vi "Untitled 1.vi"() -> ()   [LabVIEW 2025]
panel:
  out "Boolean 2":bool
  in  "Sair":bool
  out "Contador":dbl format="%#_2f"
  out "Boolean":bool
  in  "Pausar":bool
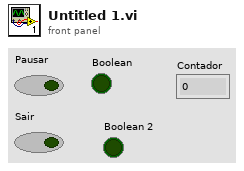
[diagram p1: front panel]
types:
  T1 = enum16{"Incializar", "Executar ", "Pausar", "Sair"}
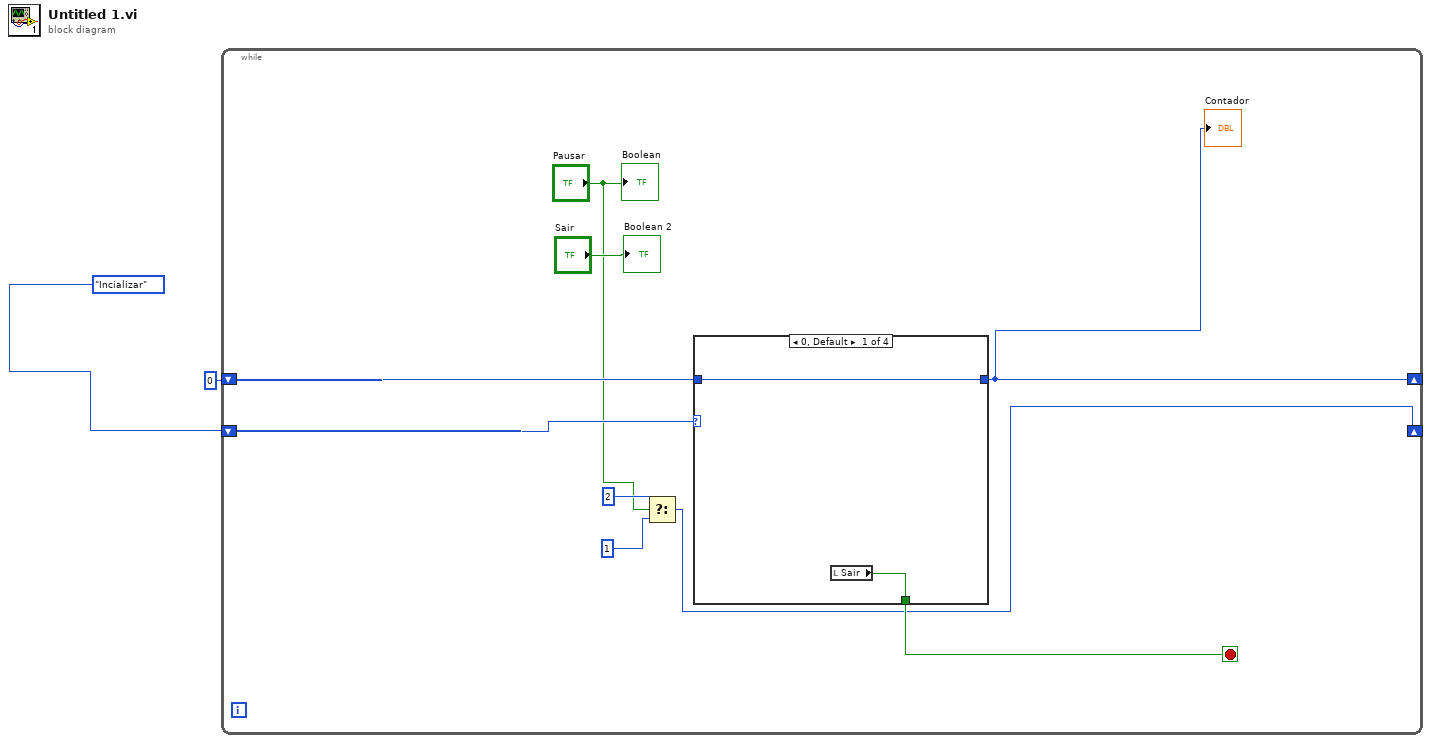
[diagram p0: block diagram]
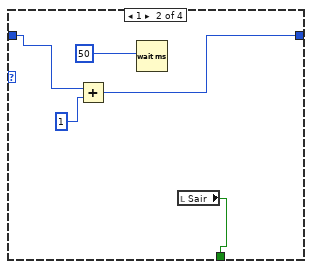
[diagram p2: hidden frame]
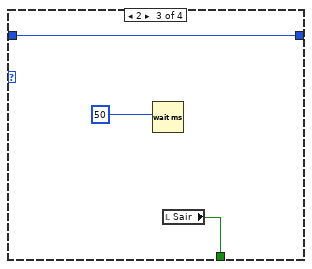
[diagram p3: hidden frame]
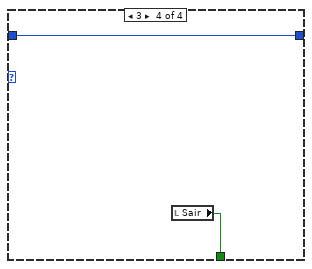
[diagram p4: hidden frame]
diagram:
  n1 = while {
    shift-right: [w7] -> _
    shift-left: 0 -> [w9]
    shift-right: [w4] -> _
    shift-left: T1."Incializar" -> [w8]
    stop <- w10 stop-if-true
    n2 = Select(t=2, s="Pausar", f=1) -> (s? t:f=w4:i32)
    n3 = case shown="0, Default" w8 {
      tunnel: [w13 w17 w21 w23] -> w10
      tunnel: w9 -> [w12 w15 w20 w22]
      tunnel: [w12 w16 w20 w22] -> w7
      frame 0, Default {
        n4 = local read "Sair"() -> (w13:bool)
      }
      frame 1 {
        n5 = Add(x=w15, y=1) -> (x+y=w16:i32)
        n6 = Wait (ms)(milliseconds to wait=50) -> ()  [unwired: 1 out]
        n7 = local read "Sair"() -> (w17:bool)
      }
      frame 2 {
        n8 = Wait (ms)(milliseconds to wait=50) -> ()  [unwired: 1 out]
        n9 = local read "Sair"() -> (w21:bool)
      }
      frame 3 {
        n10 = local read "Sair"() -> (w23:bool)
      }
    }
    "Contador" <- w7
    "Boolean" <- "Pausar"
    "Boolean 2" <- "Sair"
  }
